vi "case select tools.vi"(11 "Tool Selection":T1) -> (3 "VI out":refnum<vi>)   [LabVIEW 2016, in "main.lvlib"]
uses:
  main.lvlib
  tool selection.ctl
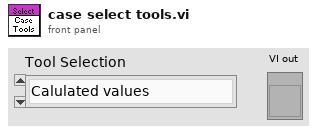
[diagram p1: front panel]
types:
  T1 = typedef "main.lvlib/tool selection.ctl" = enum16{"Calulated values", "Scale", "Currents", "Injector magnet", "Terminal Voltage", "Source BPM", "Vacuum", "Flat Top", "Zero Values", "Terminal Control", "Scan Injector"}
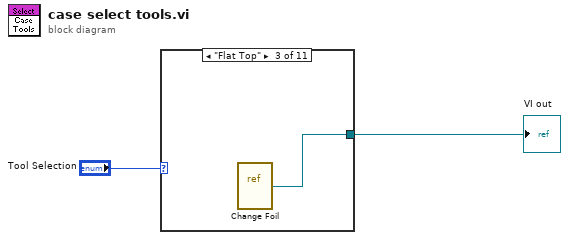
[diagram p0: block diagram]
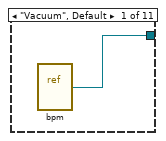
[diagram p2: hidden frame]
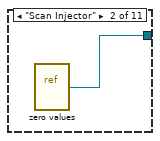
[diagram p3: hidden frame]
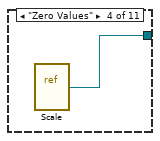
[diagram p4: hidden frame]
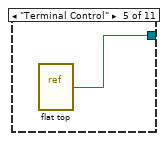
[diagram p5: hidden frame]
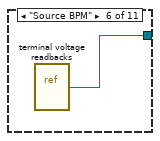
[diagram p6: hidden frame]
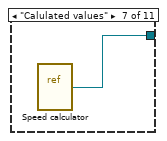
[diagram p7: hidden frame]
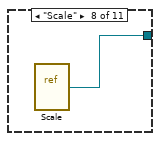
[diagram p8: hidden frame]
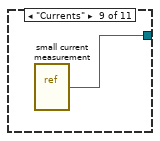
[diagram p9: hidden frame]
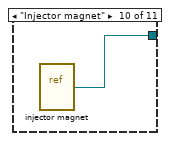
[diagram p10: hidden frame]
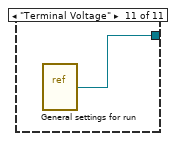
[diagram p11: hidden frame]
diagram:
  n1 = case shown="\"Flat Top\"" "Tool Selection" {
    tunnel: [w3 w4 w5 w6 w7 w8 w9 w10 w11 w12 w13] -> w1
    frame "Vacuum", Default {
      n2 = vi-ref "bpm.vi"() -> (w3:refnum<vi>)
    }
    frame "Scan Injector" {
      n3 = vi-ref "zero values.vi"() -> (w4:refnum<vi>)
    }
    frame "Flat Top" {
      n4 = vi-ref "Change Foil.vi"() -> (w5:refnum<vi>)
    }
    frame "Zero Values" {
      n5 = vi-ref "Scale.vi"() -> (w6:refnum<vi>)
    }
    frame "Terminal Control" {
      n6 = vi-ref "flat top.vi"() -> (w7:refnum<vi>)
    }
    frame "Source BPM" {
      n7 = vi-ref "terminal voltage readbacks.vi"() -> (w8:refnum<vi>)
    }
    frame "Calulated values" {
      n8 = vi-ref "Speed calculator.vi"() -> (w9:refnum<vi>)
    }
    frame "Scale" {
      n9 = vi-ref "Scale.vi"() -> (w10:refnum<vi>)
    }
    frame "Currents" {
      n10 = vi-ref "small current measurement.vi"() -> (w11:refnum<vi>)
    }
    frame "Injector magnet" {
      n11 = vi-ref "injector magnet.vi"() -> (w12:refnum<vi>)
    }
    frame "Terminal Voltage" {
      n12 = vi-ref "General settings for run.vi"() -> (w13:refnum<vi>)
    }
  }
  "VI out" <- w1
